vi "FPGA golbals.vi"() -> ()   [LabVIEW 2020]
uses:
  FPGA Typedefs/Image State.ctl
panel:
  out "MC":bool
  out "FPGA state":T1=enum."Wait N after Trigger"
  out "Encored_trigger OR Line_signal":bool
  out "Ctr_trig_signal":bool
  out "Start_acq_signal":bool
  out "Trigger In":bool
  out "Trial_signal":bool
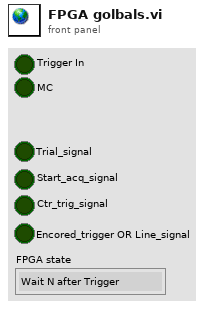
[diagram p1: front panel]
types:
  T1 = typedef "Image State.ctl" = enum16{"Start Up", "Wait for Trigger", "Wait N after Trigger", "DAQ Pointing", "DAQ Scan", "Reference Scan", "Pointing AOL Fill", "Scan AOL FILL", "Reference AOL Fill"}
diagram:
